vi "Loop Timer.vi"() -> (2 "dt":u32)   [LabVIEW 2014]
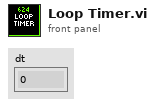
[diagram p1: front panel]
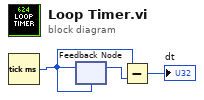
[diagram p0: block diagram]
diagram:
  n1 = Tick Count (ms)() -> (millisecond timer value=w1:u32)
  n2 = feedback-in #1(w1) -> ()
  n3 = feedback #1(w1) -> (w2:u32)
  n4 = Subtract(x=w1, y=w2) -> (x-y=→"dt":u32)
